vi "update_display_data_Init.vi"(8 "error in (no error)":errorcluster, 11 "Object in":refnum<class "update_display_data.lvclass">) -> (0 "error out":errorcluster, 3 "object out":refnum<class "update_display_data.lvclass">)   [LabVIEW 2018, in "ClientMessaging.lvlib" / "update_display_data.lvclass"]
uses:
  update_display_data.lvclass
  C:/Users/gavin/Documents/Programming/LabVIEW/JuPyterClient/IOPub Messages/display_data Message/display_data Message.lvclass
  update_display_data.lvclass/update_display_data.ctl
  display_data Message/display_data Message.lvclass
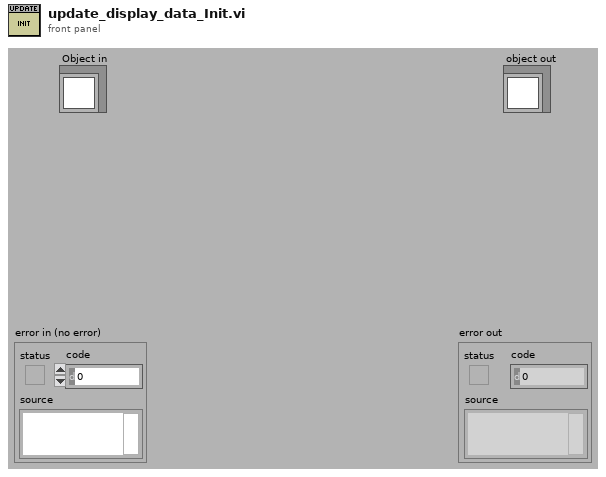
[diagram p1: front panel]
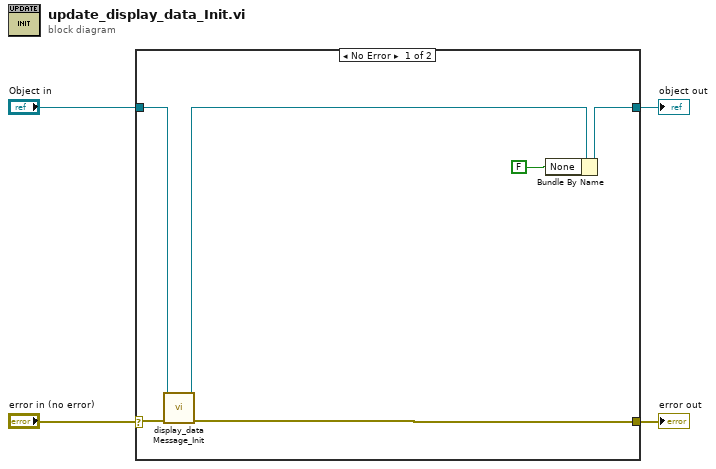
[diagram p0: block diagram]
diagram:
  n1 = case shown="No Error" "error in (no error)" {
    selector: "error in (no error)" -> [w8 w11]
    tunnel: [w10 w12] -> w4
    tunnel: "Object in" -> [w6 w12]
    tunnel: [w7 w11] -> w1
    frame No Error {
      n2 = call "display_data Message_Init.vi"("error in (no error)"=w8, "object in"=w6) -> ("error out"=w7:errorcluster, "object out"=w5:refnum<class "update_display_data.lvclass">)  [unwired: 8 in]
      n3 = Bundle By Name(cluster=w5, "None"=FALSE) -> (w10:refnum<class "update_display_data.lvclass">)
    }
    frame Error {
    }
  }
  "object out" <- w4
  "error out" <- w1
